vi "DDS States (Global).vi"() -> ()   [LabVIEW 2018]
uses:
  Controls/DDS State.ctl
panel:
  out "Gen DDS State":T1=enum."Shutdown"
  out "PCC DDS State":T1=enum."Shutdown"
  out "Load DDS State":T1=enum."Shutdown"
  out "ES_2 DDS State":T1=enum."Shutdown"
  out "ES_1 DDS State":T1=enum."Shutdown"
  out "PV DDS State":T1=enum."Shutdown"
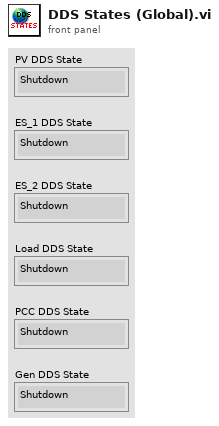
[diagram p1: front panel]
types:
  T1 = typedef "DDS State.ctl" = enum16{"Commissioning", "CheckID", "InitDDS", "ReadDDS", "WriteDDS", "CheckClose", "Close", "Shutdown"}
diagram:
